vi "ShowAllRecords.vi"(0 "reference in":refnum<class "CustomersData.lvclass">, 5 "error in (no error)":errorcluster) -> (14 "reference out":refnum<class "CustomersData.lvclass">, 19 "error out":errorcluster)   [LabVIEW 2020, in "CustomersData.lvclass"]
uses:
  CustomersData.lvclass
  C:/Projects/OpenGDS_DesignPatterns/Bridge1/DataObject_class/DataObject.lvclass
  DataObject_class/DataObject.lvclass
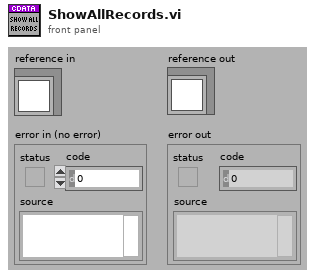
[diagram p1: front panel]
types:
  T1 = typedef "CustomersData.lvclass/ObjectAttributes.ctl" = cluster{"_customers":string[], "_current":i32}
  T2 = typedef "DataObject.lvclass/ObjectAttributes.ctl" = cluster{"StringRef":refnum<vi>}
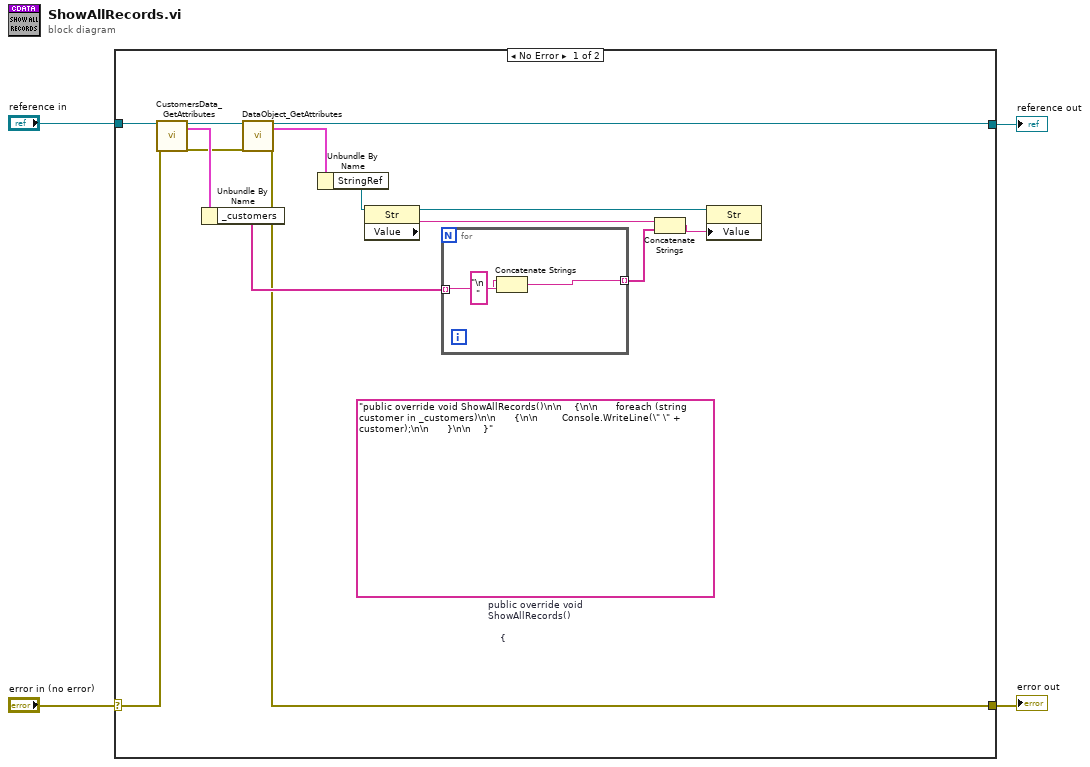
[diagram p0: block diagram]
diagram:
  n1 = case shown="No Error" "error in (no error)" {
    selector: "error in (no error)" -> [w17 w23]
    tunnel: [w5 w23] -> w3
    tunnel: [w14 w22] -> w1
    tunnel: "reference in" -> [w18 w22]
    frame No Error {
      (unwired) "public override void ShowAllRecords()\n\n    {\n\n      foreach (string customer in _customers)\n\n      {\n\n        Console.WriteLine(\" \" + customer);\n\n      }\n\n    }"  # public override void ShowAllRecords()      {        foreach (string customer in _customers)        {          Console.WriteLine(" " + customer);        }      }
      n2 = call "CustomersData_GetAttributes.vi"("reference in"=w18, "error in (no error)"=w17) -> ("reference out"=w15:refnum<class "CustomersData.lvclass">, "Data"=w16:T1, "error out"=w12:errorcluster)  [unwired: 14 in, 1 out]
      n3 = Unbundle By Name(w16) -> ("_customers"=w11:string[])
      n4 = call "DataObject_GetAttributes.vi"("reference in"=w15, "error in (no error)"=w12) -> ("reference out"=w14:refnum<class "CustomersData.lvclass">, "Data"=w13:T2, "error out"=w5:errorcluster)  [unwired: 14 in, 1 out]
      n5 = Unbundle By Name(w13) -> ("StringRef"=w10:refnum<vi>)
      n6 = property class="Str"(reference=w10) -> (reference out=w9:refnum<vi>, "Value"=w8:string)  [unwired: 1 in, 1 out]
      n7 = for {
        tunnel: w11 -> [w21] mode=indexing
        tunnel: [w19] -> w7 mode=indexing
        n8 = Concatenate Strings("\n   " ("string"), w21) -> (w19:string)
      }
      n9 = Concatenate Strings(w8, w7) -> (w6:string)
      n10 = property class="Str"(reference=w9, "Value"=w6) -> ()  [unwired: 1 in, 2 out]
    }
    frame Error {
    }
  }
  "error out" <- w3
  "reference out" <- w1
